vi "EQ choose report.vi"(0 "Chip ID list":u32[](array[numeric]) format="%.0x", 5 "quants pixels bons per Chip":u8[](array[numeric]), 7 "Folder path: EQ reports":path=path "C:/VIP Module/Files/Equalization/yyyymmdd_hh-mm-ss_Leak#_HV#", 9 "summary IDs":string, 11 "summary EQ":string) -> ()   [LabVIEW 2015, in "VIPM2.lvlib"]
doc: "Mostra en una nova finestra el resum de pixels bons per Chip.\nEn sel·leccionar una Layer, s'obre el <b>report viewer x4</b> en una segona finestra."
uses:
  VIPM2.lvlib
panel:
  in  "Choose Array":T1(array[cluster])
  in  "Close button":bool
  # "Choose one Layer to watch its report"
  # "In green, good pixels per Chip."
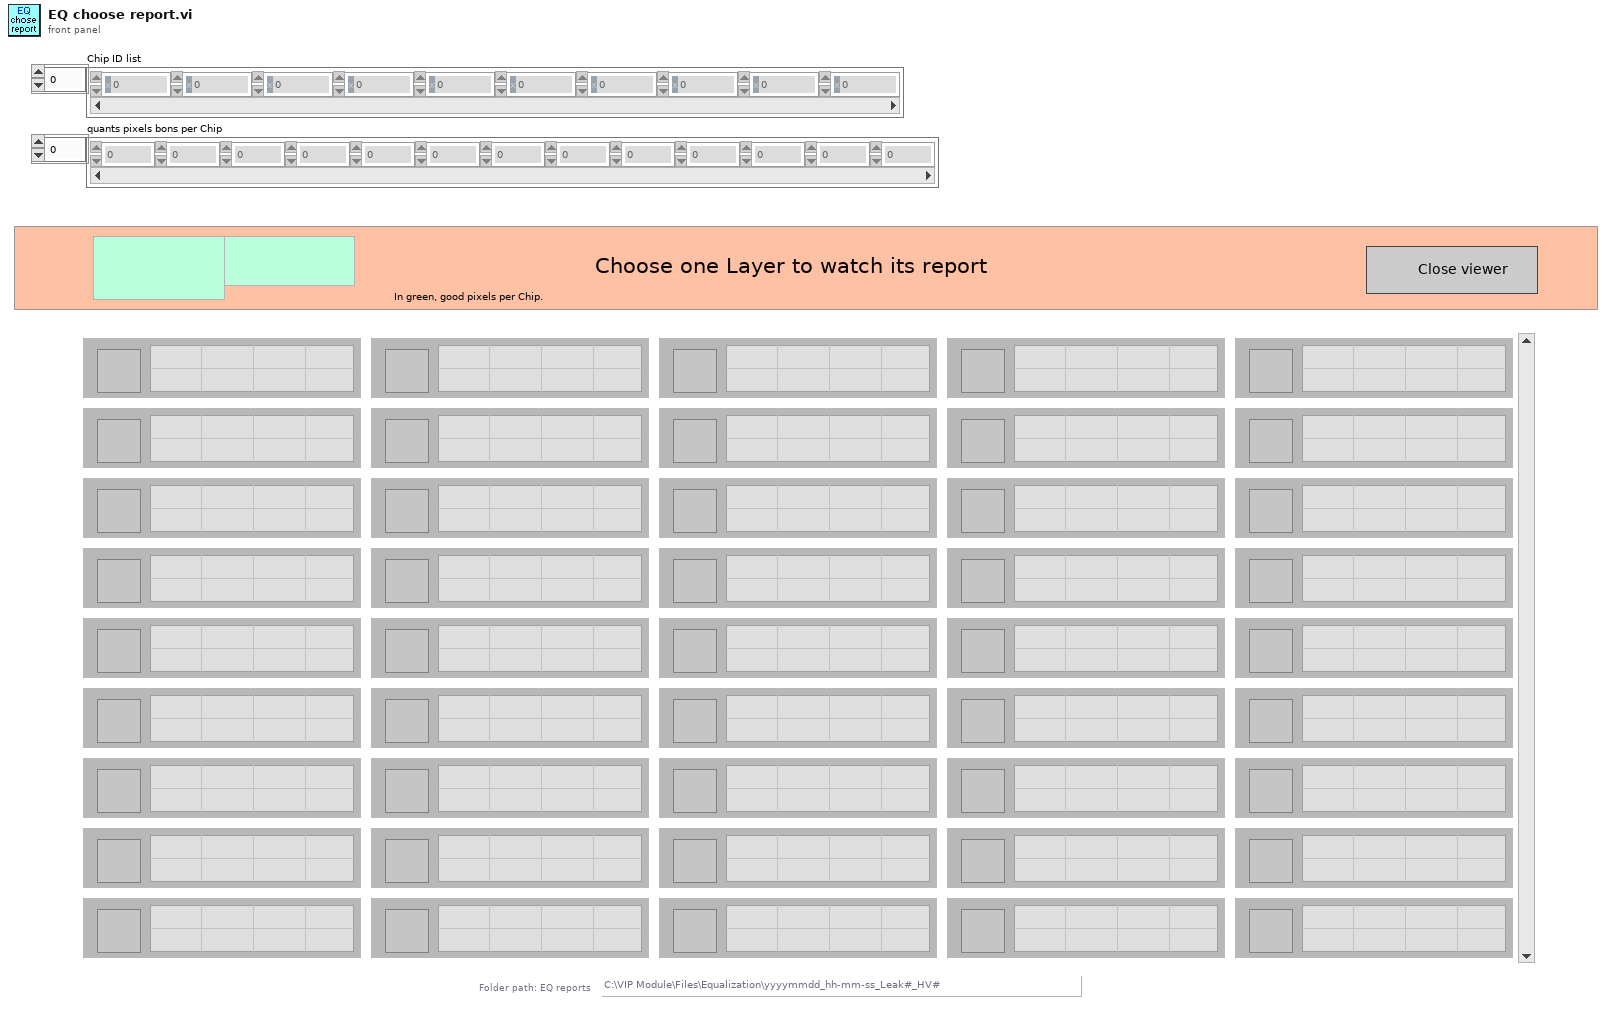
[diagram p1: front panel]
types:
  T1 = cluster{"Choose Button":bool, "Data table":string[][]}[][]
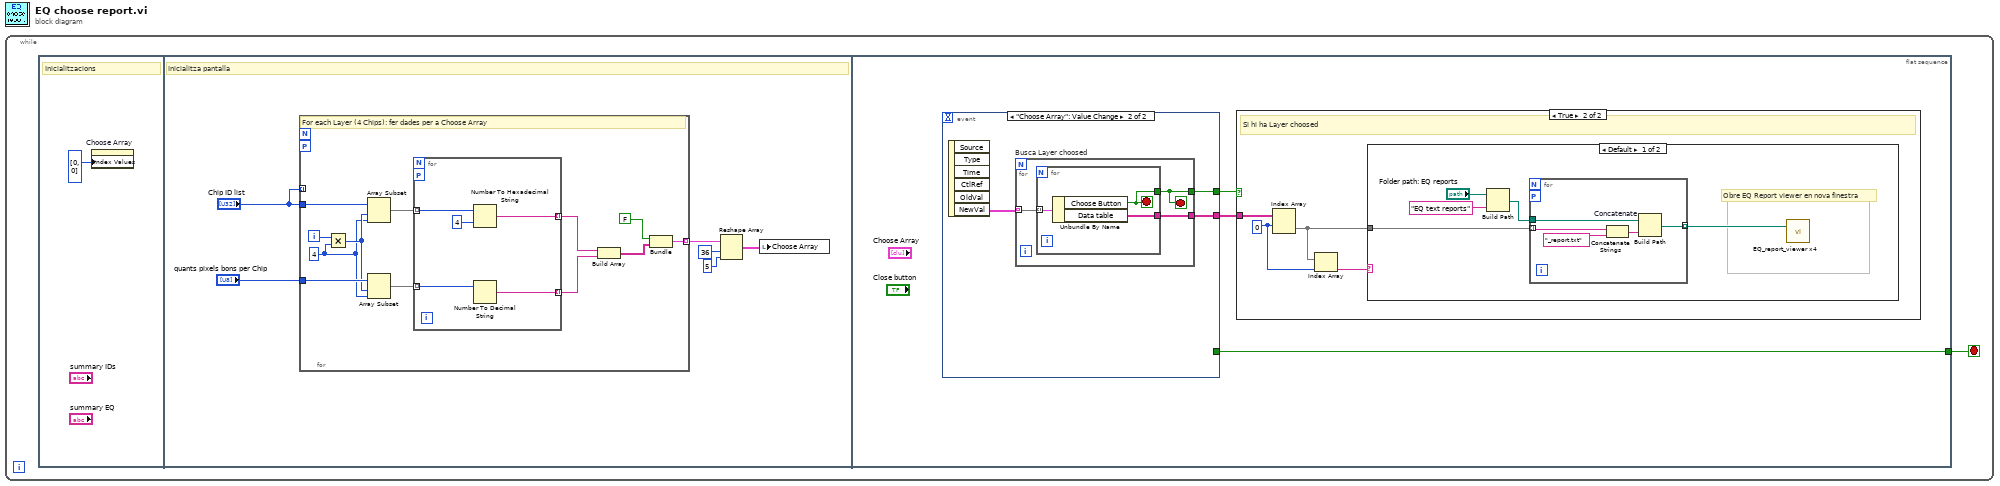
[diagram p0: block diagram]
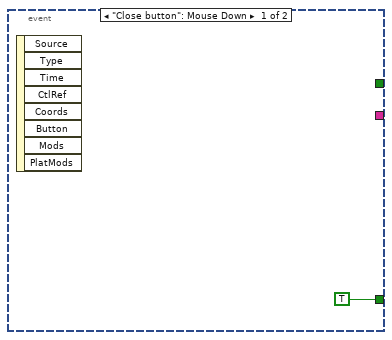
[diagram p4: hidden frame]
diagram:
  n1 = while {
    stop <- w1 stop-if-true
    n2 = flat-sequence {
      tunnel: [w26] -> w1
      frame #0 {
        # "Inicialitzacions"
        n3 = property on="Choose Array" class="Arr"("Index Values"=u32[] [0, 0]) -> ()  [unwired: 2 in, 2 out]
      }
      frame #1 {
        # "Inicialitza pantalla"
        n4 = for {
          tunnel: "Chip ID list" -> [w20]
          tunnel: "quants pixels bons per Chip" -> [w19]
          tunnel: "Chip ID list" -> [_] mode=indexing
          tunnel: [w9] -> w4 mode=indexing
          workers-P: _ -> [_]
          i -> [w18]
          w16 = 4 ("y")
          # "For each Layer (4 Chips): fer dades per a Choose Array"
          n5 = Multiply(x=w18, y=w16) -> (x*y=w17:i32)
          n6 = Array Subset "Array Subset"(array=w20, index=w17, length=w16) -> (w15:u32[])
          n7 = Array Subset(array=w19, index=w17, length=w16) -> (w14:u8[])
          n8 = for {
            tunnel: w15 -> [w25] mode=indexing
            tunnel: w14 -> [w22] mode=indexing
            tunnel: [w23] -> w13 mode=indexing
            tunnel: [w21] -> w12 mode=indexing
            workers-P: _ -> [_]
            n9 = Number To Hexadecimal String(1:i16 4 ("width (-)"), 2:w25) -> (0:w23:string)
            n10 = Number To Decimal String(number=w22) -> (decimal integer string=w21:string)  [unwired: 1 in]
          }
          n11 = Build Array "Build Array"(w13, w12) -> (w10:string[][])
          n12 = Bundle("Choose Button"=FALSE, w10) -> (w9:cluster{"Choose Button":bool, string[][]})  [unwired: 1 in]
        }
        n13 = Reshape Array "Reshape Array"(w4, 36 ("dimension size"), 5 ("dimension size")) -> (w3:cluster{"Choose Button":bool, string[][]}[][])
        n14 = local write "Choose Array"(w3) -> ()
      }
      frame #2 {
        n15 = event shown="[1] \"Choose Array\": Value Change" {
          selector: _ -> [_ _]
          dyn-events: _ -> [_ _]
          timeout: _ -> [_ _]
          tunnel: [TRUE _] -> w26
          tunnel: [_ w45] -> w28
          tunnel: [_ w44] -> w27
          event "Close button": Mouse Down {
            n16 = event-data() -> ()  [unwired: 1 in, 8 out]
          }
          event "Choose Array": Value Change {
            n17 = event-data() -> ("NewVal"=w46:T1)  [unwired: 1 in, 5 out]
            n18 = for "Busca Layer choosed" {
              tunnel: w46 -> [w49] mode=indexing
              tunnel: [w48] -> w44
              tunnel: [w47] -> w45
              stop <- w47 stop-if-true
              n19 = for {
                tunnel: w49 -> [w52] mode=indexing
                tunnel: [w51] -> w48
                tunnel: [w50] -> w47
                stop <- w50 stop-if-true
                n20 = Unbundle By Name(w52) -> ("Choose Button"=w50:bool, "Data table"=w51:string[][])
              }
            }
          }
        }
        n21 = case shown="True" w28 {
          tunnel: w27 -> [_ w32]
          frame False {
            # "choosed no vàlid"
          }
          frame True {
            w31 = 0 ("index (row)")
            # "Si hi ha Layer choosed"
            n22 = Index Array "Index Array"(array=w32, index (row)=w31) -> (element=w29:string[])  [unwired: 1 in]
            n23 = Index Array "Index Array"(array=w29, index=w31) -> (element=w30:string)
            n24 = case shown="Default" w30 {
              tunnel: w29 -> [w36 _]
              frame Default {
                # "Obre EQ Report viewer en nova finestra"
                n25 = Build Path(base path="Folder path: EQ reports", name or relative path="EQ text reports") -> (appended path=w35:path)
                n26 = for {
                  tunnel: w36 -> [w40] mode=indexing
                  tunnel: w35 -> [w39]
                  tunnel: [w38] -> w34 mode=indexing
                  workers-P: _ -> [_]
                  n27 = Concatenate Strings "Concatenate"(w40, "_report.txt" ("substring (\"\")")) -> (w42:string)
                  n28 = Build Path(base path=w39, name or relative path=w42) -> (appended path=w38:path)
                }
                n29 = call "EQ_report_viewer x4.vi"("folder path"=w34) -> ()  [unwired: 2 in]
              }
              frame "" {
                # "empty array: choose another"
              }
            }
          }
        }
      }
    }
  }
